vi "启动条件判断.vi"(8 "仪器状态":bool, 9 "启动次数":i32, 10 "间隔计时":i32, 11 "周期设置输出":T4 {"定点周期"."启动命令 24" items=["", "水样测试", "标样核查", "零点核查", "跨度核查", "空白测试", "平行样测试", "加标回收", "空白校准", "标样校准"]; "定点周期"."启动命令 23" items=["", "水样测试", "标样核查", "零点核查", "跨度核查", "空白测试", "平行样测试", "加标回收", "空白校准", "标样校准"]; "定点周期"."启动命令 22" items=["", "水样测试", "标样核查", "零点核查", "跨度核查", "空白测试", "平行样测试", "加标回收", "空白校准", "标样校准"]; "定点周期"."启动命令 21" items=["", "水样测试", "标样核查", "零点核查", "跨度核查", "空白测试", "平行样测试", "加标回收", "空白校准", "标样校准"]; "定点周期"."启动命令 20" items=["", "水样测试", "标样核查", "零点核查", "跨度核查", "空白测试", "平行样测试", "加标回收", "空白校准", "标样校准"]; "定点周期"."启动命令 19" items=["", "水样测试", "标样核查", "零点核查", "跨度核查", "空白测试", "平行样测试", "加标回收", "空白校准", "标样校准"]; "定点周期"."启动命令 18" items=["", "水样测试", "标样核查", "零点核查", "跨度核查", "空白测试", "平行样测试", "加标回收", "空白校准", "标样校准"]; "定点周期"."启动命令 17" items=["", "水样测试", "标样核查", "零点核查", "跨度核查", "空白测试", "平行样测试", "加标回收", "空白校准", "标样校准"]; "定点周期"."启动命令 16" items=["", "水样测试", "标样核查", "零点核查", "跨度核查", "空白测试", "平行样测试", "加标回收", "空白校准", "标样校准"]; "定点周期"."启动命令 15" items=["", "水样测试", "标样核查", "零点核查", "跨度核查", "空白测试", "平行样测试", "加标回收", "空白校准", "标样校准"]; "定点周期"."启动命令 14" items=["", "水样测试", "标样核查", "零点核查", "跨度核查", "空白测试", "平行样测试", "加标回收", "空白校准", "标样校准"]; "定点周期"."启动命令 13" items=["", "水样测试", "标样核查", "零点核查", "跨度核查", "空白测试", "平行样测试", "加标回收", "空白校准", "标样校准"]; "定点周期"."启动命令 12" items=["", "水样测试", "标样核查", "零点核查", "跨度核查", "空白测试", "平行样测试", "加标回收", "空白校准", "标样校准"]; "定点周期"."启动命令 11" items=["", "水样测试", "标样核查", "零点核查", "跨度核查", "空白测试", "平行样测试", "加标回收", "空白校准", "标样校准"]; "定点周期"."启动命令 10" items=["", "水样测试", "标样核查", "零点核查", "跨度核查", "空白测试", "平行样测试", "加标回收", "空白校准", "标样校准"]; "定点周期"."启动命令 9" items=["", "水样测试", "标样核查", "零点核查", "跨度核查", "空白测试", "平行样测试", "加标回收", "空白校准", "标样校准"]; "定点周期"."启动命令 8" items=["", "水样测试", "标样核查", "零点核查", "跨度核查", "空白测试", "平行样测试", "加标回收", "空白校准", "标样校准"]; "定点周期"."启动命令 7" items=["", "水样测试", "标样核查", "零点核查", "跨度核查", "空白测试", "平行样测试", "加标回收", "空白校准", "标样校准"]; "定点周期"."启动命令 6" items=["", "水样测试", "标样核查", "零点核查", "跨度核查", "空白测试", "平行样测试", "加标回收", "空白校准", "标样校准"]; "定点周期"."启动命令 5" items=["", "水样测试", "标样核查", "零点核查", "跨度核查", "空白测试", "平行样测试", "加标回收", "空白校准", "标样校准"]; "定点周期"."启动命令 4" items=["", "水样测试", "标样核查", "零点核查", "跨度核查", "空白测试", "平行样测试", "加标回收", "空白校准", "标样校准"]; "定点周期"."启动命令 3" items=["", "水样测试", "标样核查", "零点核查", "跨度核查", "空白测试", "平行样测试", "加标回收", "空白校准", "标样校准"]; "定点周期"."启动命令 2" items=["", "水样测试", "标样核查", "零点核查", "跨度核查", "空白测试", "平行样测试", "加标回收", "空白校准", "标样校准"]; "定点周期"."启动命令" items=["", "水样测试", "标样核查", "零点核查", "跨度核查", "空白测试", "平行样测试", "加标回收", "空白校准", "标样校准"]; "间隔设置"."启动命令" items=["", "水样测试", "标样核查", "零点核查", "跨度核查", "空白测试", "平行样测试", "加标回收", "空白校准", "标样校准"]}) -> (2 "重新配置":bool, 3 "Data":T5 caption="数据")   [LabVIEW 2016, in "定时设置.xctl"]
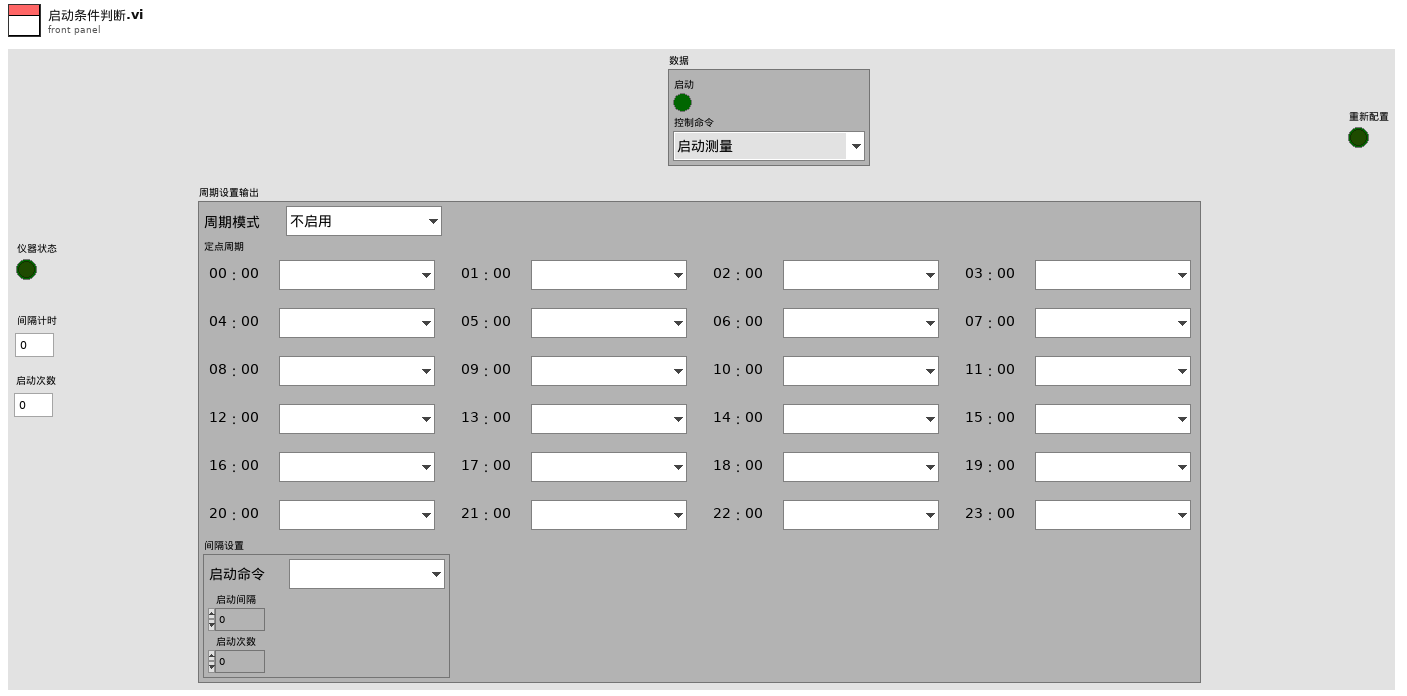
[diagram p1: front panel]
types:
  T1 = typedef "定时设置.xctl/周期模式设置.ctl" = enum16{"不启用", "定点模式", "间隔模式"}
  T2 = typedef "定时设置.xctl/定点周期设置.ctl" = cluster{"启动命令":T3, "启动命令 2":T3, "启动命令 3":T3, "启动命令 4":T3, "启动命令 5":T3, "启动命令 6":T3, "启动命令 7":T3, "启动命令 8":T3, "启动命令 9":T3, "启动命令 10":T3, "启动命令 11":T3, "启动命令 12":T3, "启动命令 13":T3, "启动命令 14":T3, "启动命令 15":T3, "启动命令 16":T3, "启动命令 17":T3, "启动命令 18":T3, "启动命令 19":T3, "启动命令 20":T3, "启动命令 21":T3, "启动命令 22":T3, "启动命令 23":T3, "启动命令 24":T3}
  T3 = typedef "定时设置.xctl/启动命令选择.ctl" = u16
  T4 = cluster{"周期模式":T1, "定点周期":T2, "间隔设置":cluster{"启动命令":T3, "启动间隔":dbl, "启动次数":i32}}
  T5 = typedef "定时设置.xctl/数据.ctl" = cluster{"启动":bool, "控制命令":T6}
  T6 = typedef "定时设置.xctl/国标控制命令.ctl" = enum16{"启动测量", "标样核查", "零点核查", "跨度核查", "空白测试", "平行样测试", "加标回收", "空白校准", "标样校准", "初始化（清洗）", "停止测试", "仪器重启", "校时", "模式设置", "测量间隔设置"}
  T7 = typedef "LVDateTimeRec.ctl" = cluster{"秒数的小数部分":dbl, "秒":i32, "分":i32, "时":i32, "日":i32, "月":i32, "年":i32, "天数（周）":i32, "天数（年）":i32, "DST":i32}
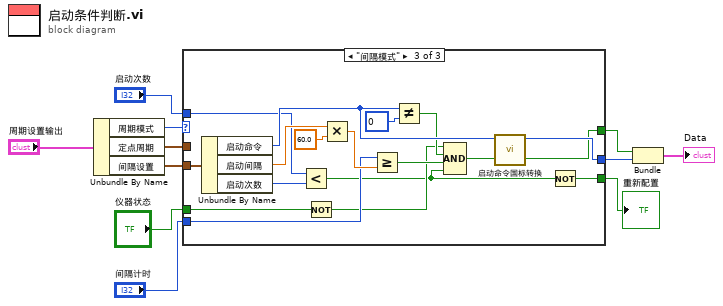
[diagram p0: block diagram]
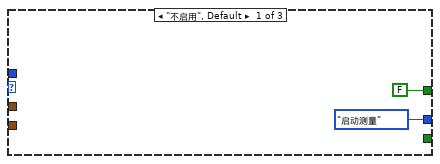
[diagram p2: hidden frame]
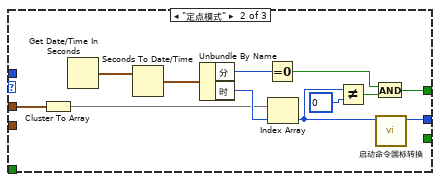
[diagram p3: hidden frame]
diagram:
  n1 = Unbundle By Name("周期设置输出") -> ("周期模式"=w11:T1, "定点周期"=w10:T2, "间隔设置"=w9:cluster{"启动命令":T3, "启动间隔":dbl, "启动次数":i32})
  n2 = case shown="\"间隔模式\"" w11 {
    tunnel: w10 -> [_ w15 _]
    tunnel: w9 -> [_ _ w42]
    tunnel: [国标控制命令."启动测量" ("控制命令") w17 w41] -> w7
    tunnel: [FALSE w16 w32] -> w2
    tunnel: "启动次数" -> [_ _ w36]
    tunnel: "间隔计时" -> [_ _ w30]
    tunnel: "仪器状态" -> [_ _ w29]
    tunnel: [_ _ w26] -> w1
    frame "不启用", Default {
    }
    frame "定点模式" {
      w22 = T3 0 items=["", "水样测试", "标样核查", "零点核查", "跨度核查", "空白测试", "平行样测试", "加标回收", "空白校准", "标样校准"] ("y")
      n3 = Cluster To Array(cluster=w15) -> (array=w14:T3[])
      n4 = Get Date/Time In Seconds() -> (seconds since 1Jan1904=w25:timestamp)
      n5 = Seconds To Date/Time(time stamp (now)=w25) -> (date time rec=w24:T7)  [unwired: 1 in]
      n6 = Unbundle By Name(w24) -> ("分"=w21:i32, "时"=w23:i32)
      n7 = Equal To 0?(x=w21) -> (x = 0?=w19:bool)
      n8 = Index Array(array=w14, index=w23) -> (element=w18:T3)
      n9 = Not Equal?(x=w18, y=w22) -> (x != y?=w20:bool)
      n10 = And(x=w19, y=w20) -> (x .and. y?=w16:bool)
      n11 = call "启动命令国标转换.vi"("启动命令"=w18) -> ("控制命令"=w17:T6)  [unwired: 10 in]
    }
    frame "间隔模式" {
      w39 = T3 0 items=["", "水样测试", "标样核查", "零点核查", "跨度核查", "空白测试", "平行样测试", "加标回收", "空白校准", "标样校准"] ("y")
      n12 = Unbundle By Name(w42) -> ("启动命令"=w40:T3, "启动间隔"=w38:dbl, "启动次数"=w35:i32)
      n13 = Less?(x=w36, y=w35) -> (x < y?=w27:bool)
      n14 = Not(x=w29) -> (.not. x?=w28:bool)
      n15 = Multiply(x=w38, y=60.0) -> (x*y=w31:dbl)
      n16 = Greater Or Equal?(x=w30, y=w31) -> (x >= y?=w33:bool)
      n17 = Not Equal?(x=w40, y=w39) -> (x != y?=w34:bool)
      n18 = Compound Arithmetic op=AND ("复合运算")(w28, w34, w33, w27) -> (w32:bool)
      n19 = call "启动命令国标转换.vi"("启动命令"=w40) -> ("控制命令"=w41:T6)  [unwired: 10 in]
      n20 = Not(x=w27) -> (.not. x?=w26:bool)
    }
  }
  "重新配置" <- w1
  n21 = Bundle(w2, "控制命令"=w7) -> (→"Data":cluster{bool, "控制命令":T6})  [unwired: 1 in]
